vi "Digital_IO.vi"(2 "error in":errorcluster, 3 "Data in":string) -> (0 "error out (no error)":errorcluster)   [LabVIEW 2011]
doc: "Digital IO Control vi.\n\nThe Digital_IO_Control control the basic input and output to and from USB. \n\n<Function><...>\n\nFunction Enum (Integer)\nClear all cards 1\nClear multiple cards 3\nBuild a complete card 9\n\nClear all cards:\nClear all relays on all cards.\n\nClear multiple cards: <Card mask>\nClear all relays multiple cards.\n\n<Card> : Integer\nWhich cards to clear.\n\nBuild a complete card: <Card><Data>\n\n<Card> : Integer\nWhich card to build a row on.\n\n<Data> : Integer\nDescribes which relay(s) on a card to enable."
uses:
  Server_Globals.vi
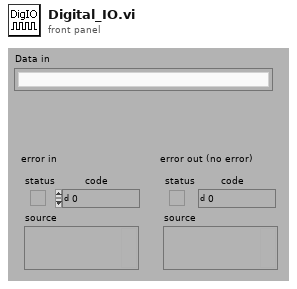
[diagram p1: front panel]
types:
  T1 = cluster{"I/O Settings":u64[], "Instrument Handle":cluster{"5402":refnum<k15>, " 5112":refnum<k15>, "4072":refnum<k15>, "USB":refnum<visa-resource-name>, "4110":refnum<k15>}, "Logfile":refnum<file>, "Log Level":i8, "Clear":i32[], "OS Set":cluster{"instrument handle out":refnum<k15>, "remaining string":string, "Settings":cluster{"Horizontal Conf.":cluster{"Min. Sample rate":dbl, "Reference position":dbl, "Record Length":i16}, "Channel A":cluster{"Enable":bool, "Vertical coupling":dbl, "Vertical range":dbl, "Vertical offset":dbl, "Probe attenuation":dbl}, "Channel B":cluster{"Enable":bool, "Vertical coupling":dbl, "Vertical range":dbl, "Vertical offset":dbl, "Probe attenuation":dbl}, "Trigger":cluster{"Source":enum8{"channel 1", "channel 2", "Imediate", "External trigger"}, "Slope":enum8{"Positive", "Negative"}, "Coupling":enum8{"AC", "DC"}, "Level":dbl, "Holdoff":dbl, "Delay":dbl, " Timeout":dbl, " Mode":enum8{"Normal", "Auto", "Auto Level"}}, "Measurements":cluster{"Measurement 1, Channel":enum8{"Channel 1", "Channel 2", "Channel 3", "Channel 4"}, "Measurement 1, Selection":u16, "Measurement 2, Channel":enum8{"Channel 1", "Channel 2", "Channel 3", "Channel 4"}, "Measurement 2,  Selection":u16, "Measurement 3, Channel":enum8{"Channel 1", "Channel 2", "Channel 3", "Channel 4"}, "Measurement 3, Selection 3":u16}}}, "DC Power Supply":cluster{"0":refnum<k15>, "1":refnum<k15>, "2":refnum<k15>, "3":refnum<k15>, "4":refnum<k15>}, "USB Interface":cluster{"0":refnum<visa-resource-name>, "1":refnum<visa-resource-name>, "2":refnum<visa-resource-name>, "3":refnum<visa-resource-name>, "4":refnum<visa-resource-name>}, "Function Generator":cluster{"0":refnum<k15>, "1":refnum<k15>, "2":refnum<k15>, "3":refnum<k15>, "4":refnum<k15>}, "Digital Multimeter":cluster{"0":refnum<k15>, "1":refnum<k15>, "2":refnum<k15>, "3":refnum<k15>, "4":refnum<k15>}, "Digital Osciliscope":cluster{"0":refnum<k15>, "1":refnum<k15>, "2":refnum<k15>, "3":refnum<k15>, "4":refnum<k15>}, "To M Server":string, "Adres":string[][], "Matrix version":string, "MD5":string, "Digital Multimeter Card 2":cluster{"0":string, "1":string, "2":string, "3":string, "4":string}}
  T2 = cluster{"0":refnum<visa-resource-name>, "1":refnum<visa-resource-name>, "2":refnum<visa-resource-name>, "3":refnum<visa-resource-name>, "4":refnum<visa-resource-name>}
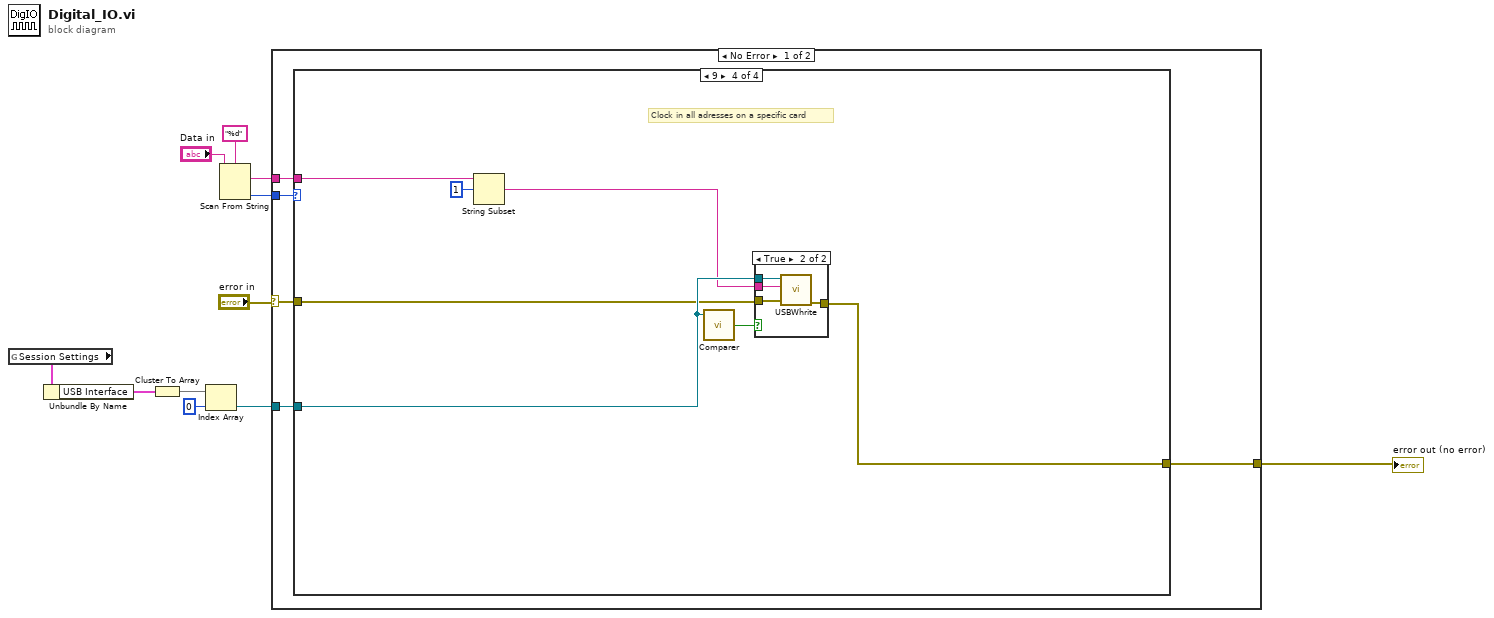
[diagram p0: block diagram]
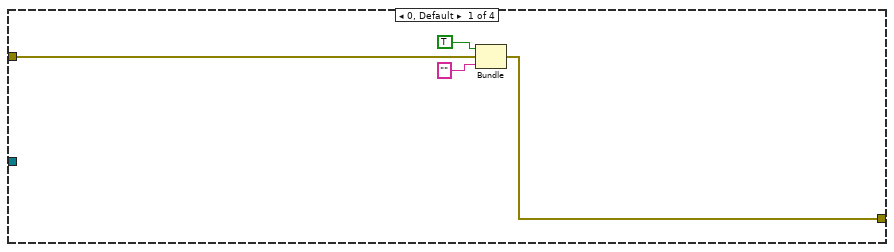
[diagram p2: hidden frame]
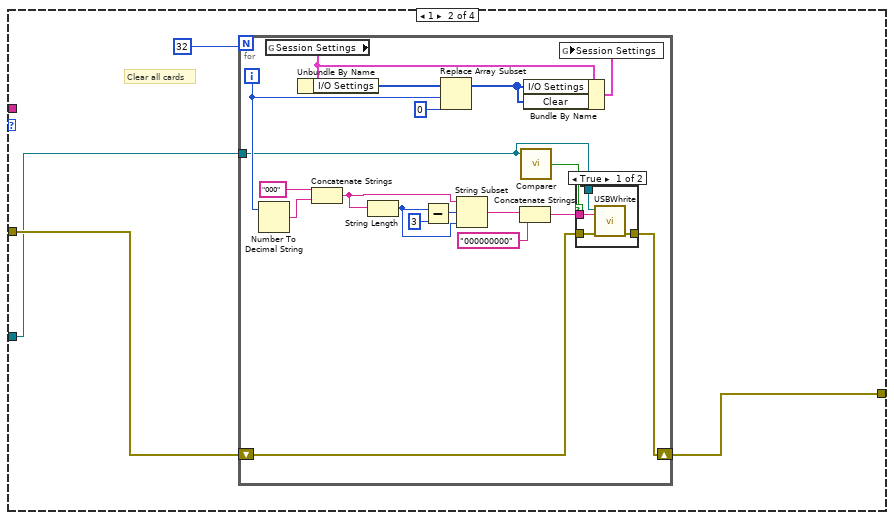
[diagram p3: hidden frame]
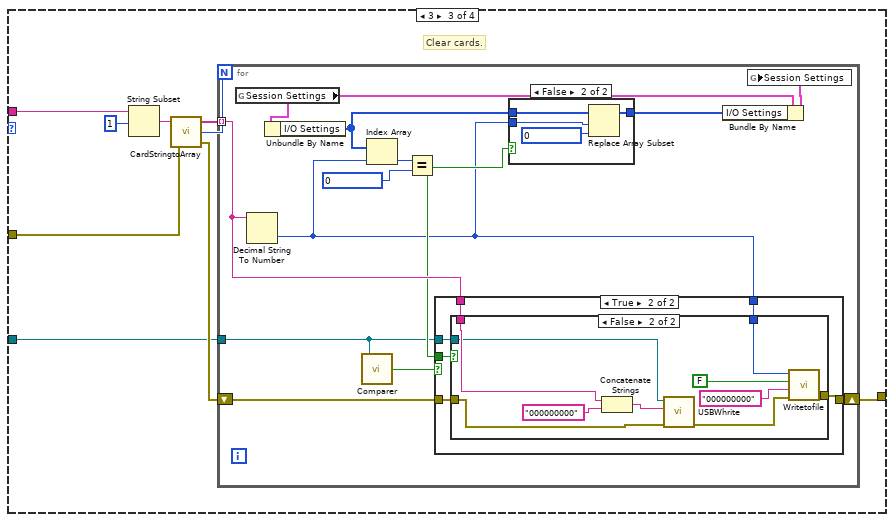
[diagram p5: hidden frame]
diagram:
  n1 = global read "Server_Globals.vi" "Session Settings"() -> (w6:T1)
  n2 = Unbundle By Name(w6) -> ("USB Interface"=w5:T2)
  n3 = Cluster To Array(cluster=w5) -> (array=w4:refnum<visa-resource-name>[])
  n4 = Index Array(array=w4, index=0) -> (element=w2:refnum<visa-resource-name>)
  n5 = Scan From String(format string="%d", input string="Data in") -> (remaining string=w7:string, output 1=w8:i32)  [unwired: 3 in, 2 out]
  n6 = case shown="No Error" "error in" {
    selector: "error in" -> [w16 w106]
    tunnel: [w13 w106] -> w1
    tunnel: w7 -> [w15 _]
    tunnel: w8 -> [w14 _]
    tunnel: w2 -> [w12 _]
    frame No Error {
      n7 = case shown="9" w14 {
        tunnel: [w19 w22 w53 w98] -> w13
        tunnel: w16 -> [w20 w23 w56 w96]
        tunnel: w15 -> [_ _ w52 w100]
        tunnel: w12 -> [_ w21 w49 w97]
        frame 0, Default {
          n8 = Bundle(cluster=w20, "status"=TRUE, "source"="") -> (w19:errorcluster)  [unwired: 1 in]
        }
        frame 1 {
          # "Clear all cards"
          n9 = for {
            N: 32 -> [_]
            shift-right: [w27] -> w22
            shift-left: w23 -> [w28]
            tunnel: w21 -> [w25]
            i -> [w32]
            n10 = Number To Decimal String(number=w32) -> (decimal integer string=w43:string)  [unwired: 1 in]
            n11 = global read "Server_Globals.vi" "Session Settings"() -> (w34:T1)
            n12 = Unbundle By Name(w34) -> ("I/O Settings"=w33:u64[])
            n13 = Concatenate Strings("000", w43) -> (w41:string)
            n14 = String Length(string=w41) -> (length=w38:i32)
            n15 = Subtract(x=w38, y=3) -> (x-y=w40:i32)
            n16 = Replace Array Subset(array=w33, new element=0, index=w32) -> (w30:u64[])
            n17 = String Subset(string=w41, offset (0)=w40, length (rest)=w38) -> (substring=w37:string)
            n18 = Concatenate Strings(w37, "000000000") -> (w29:string)
            n19 = call "Comparer.vi"("Resource name"=w25) -> ("Boolean"=w26:bool)  [unwired: 3 in, 1 out]
            n20 = Bundle By Name(cluster=w34, "I/O Settings"=w30, "Clear"=w30) -> (w35:T1)
            n21 = global write "Server_Globals.vi" "Session Settings"(w35) -> ()
            n22 = case shown="True" w26 {
              tunnel: w29 -> [w47 _]
              tunnel: w28 -> [w46 w48]
              tunnel: [w45 w48] -> w27
              tunnel: w25 -> [w44 _]
              frame True {
                n23 = call "USBWhrite.vi"("error in (no error)"=w46, "Bulk Out Data:"=w47, "USB"=w44) -> ("error out"=w45:errorcluster)  [unwired: 7 in, 1 out]
              }
              frame False {
              }
            }
          }
        }
        frame 3 {
          # "Clear cards."
          n24 = String Subset(string=w52, offset (0)=1) -> (substring=w51:string)  [unwired: 1 in]
          n25 = call "CardStringtoArray.vi"("error in (no error)"=w56, "Card In"=w51) -> ("error out"=w54:errorcluster, "N:r Cards"=w57:i32, "Card Array"=w55:string[])  [unwired: 1 in]
          n26 = for {
            N: w57 -> [_]
            tunnel: w55 -> [w67] mode=indexing
            shift-right: [w60] -> w53
            shift-left: w54 -> [w66]
            tunnel: w49 -> [w58]
            n27 = global read "Server_Globals.vi" "Session Settings"() -> (w69:T1)
            n28 = Decimal String To Number(string=w67) -> (number=w61:i32)  [unwired: 2 in, 1 out]
            n29 = Unbundle By Name(w69) -> ("I/O Settings"=w65:u64[])
            n30 = call "Comparer.vi"("Resource name"=w58) -> ("Boolean"=w59:bool)  [unwired: 3 in, 1 out]
            n31 = Index Array(array=w65, index=w61) -> (element=w64:u64)
            n32 = Equal?(x=w64, y=0) -> (x = y?=w62:bool)
            n33 = case shown="True" w59 {
              tunnel: w67 -> [_ w77]
              tunnel: w66 -> [w71 w76]
              tunnel: w62 -> [_ w75]
              tunnel: w61 -> [_ w74]
              tunnel: w58 -> [_ w73]
              tunnel: [w71 w72] -> w60
              frame False {
              }
              frame True {
                n34 = case shown="False" w75 {
                  tunnel: [w78 w88] -> w72
                  tunnel: w77 -> [_ w86]
                  tunnel: w76 -> [w78 w82]
                  tunnel: w74 -> [_ w80]
                  tunnel: w73 -> [_ w79]
                  frame True {
                  }
                  frame False {
                    n35 = Concatenate Strings(w86, "000000000") -> (w83:string)
                    n36 = call "USBWhrite.vi"("error in (no error)"=w82, "Bulk Out Data:"=w83, "USB"=w79) -> ("error out"=w81:errorcluster)  [unwired: 7 in, 1 out]
                    n37 = call "Writetofile.vi"("error in (no error)"=w81, "Componenet"="000000000", "Write"=FALSE, "Card"=w80) -> ("error out"=w88:errorcluster)  [unwired: 2 in]
                  }
                }
              }
            }
            n38 = case shown="False" w62 {
              tunnel: [w89 w93] -> w68
              tunnel: w65 -> [w89 w91]
              tunnel: w61 -> [_ w90]
              frame True {
              }
              frame False {
                n39 = Replace Array Subset(array=w91, new element=0, index=w90) -> (w93:u64[])
              }
            }
            n40 = Bundle By Name(cluster=w69, "I/O Settings"=w68) -> (w70:T1)
            n41 = global write "Server_Globals.vi" "Session Settings"(w70) -> ()
          }
        }
        frame 9 {
          # "Clock in all adresses on a specific card"
          n42 = String Subset(string=w100, offset (0)=1) -> (substring=w95:string)  [unwired: 1 in]
          n43 = call "Comparer.vi"("Resource name"=w97) -> ("Boolean"=w94:bool)  [unwired: 3 in, 1 out]
          n44 = case shown="True" w94 {
            tunnel: w96 -> [w101 w105]
            tunnel: w95 -> [_ w104]
            tunnel: [w101 w103] -> w98
            tunnel: w97 -> [_ w102]
            frame False {
            }
            frame True {
              n45 = call "USBWhrite.vi"("error in (no error)"=w105, "Bulk Out Data:"=w104, "USB"=w102) -> ("error out"=w103:errorcluster)  [unwired: 7 in, 1 out]
            }
          }
        }
      }
    }
    frame Error {
      # "An error has occoured prior to this control."
    }
  }
  "error out (no error)" <- w1
